vi "sub_ofdm_subcarrier_allocator.vi"(8 "fft size":i32=256, 9 "pilot symbol":cdb[](array[numeric]), 11 "message symbol":cdb[](array[numeric])) -> (3 "OFDM symbol":cdb[](array[numeric]))   [LabVIEW 2014]
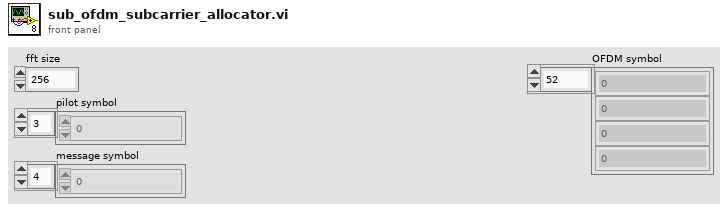
[diagram p1: front panel]
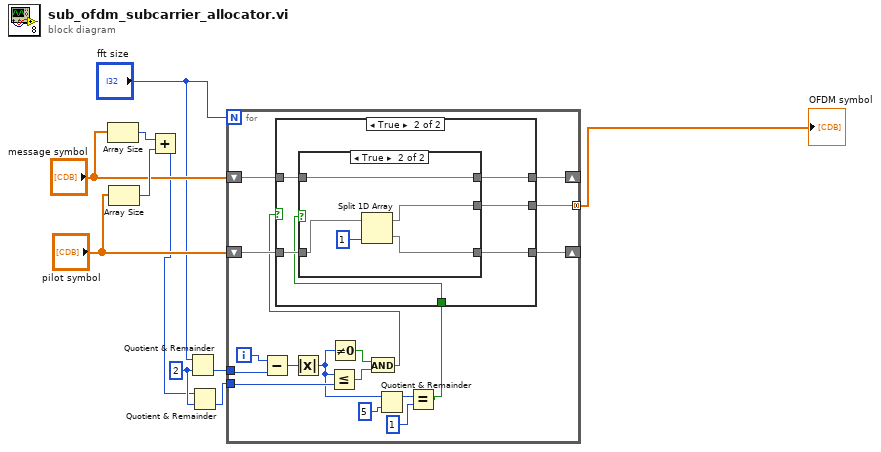
[diagram p0: block diagram]
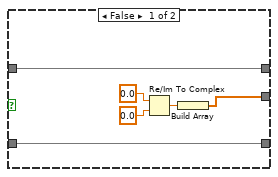
[diagram p2: hidden frame]
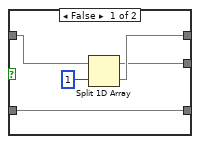
[diagram p3: hidden frame]
diagram:
  w3 = 2
  n1 = Array Size(array="message symbol") -> (size(s)=w10:i32)
  n2 = Array Size(array="pilot symbol") -> (size(s)=w9:i32)
  n3 = Add(x=w10, y=w9) -> (x+y=w2:i32)
  n4 = Quotient & Remainder(x="fft size", y=w3) -> (floor(x/y)=w5:i32)  [unwired: 1 out]
  n5 = Quotient & Remainder(x=w2, y=w3) -> (floor(x/y)=w1:i32)  [unwired: 1 out]
  n6 = for {
    N: "fft size" -> [_]
    shift-right: [w26] -> _
    shift-left: "pilot symbol" -> [w27]
    shift-right: [w20] -> _
    shift-left: "message symbol" -> [w25]
    tunnel: [w24] -> w4 mode=concatenating
    tunnel: w5 -> [w22]
    tunnel: w1 -> [w19]
    i -> [w23]
    n7 = Subtract(x=w23, y=w22) -> (x-y=w21:i32)
    n8 = Absolute Value(x=w21) -> (abs(x)=w15:i32)
    n9 = Less Or Equal?(x=w15, y=w19) -> (x <= y?=w17:bool)
    n10 = Not Equal To 0?(x=w15) -> (x != 0?=w18:bool)
    n11 = And(x=w18, y=w17) -> (x .and. y?=w16:bool)
    n12 = Quotient & Remainder(x=w15, y=5) -> (x-y*floor(x/y)=w13:i32)  [unwired: 1 out]
    n13 = Equal?(x=w13, y=1) -> (x = y?=w12:bool)
    n14 = case shown="True" w16 {
      tunnel: w27 -> [w32 w39]
      tunnel: [w32 w38] -> w26
      tunnel: w25 -> [w33 w37]
      tunnel: [w28 w36] -> w24
      tunnel: [w33 w35] -> w20
      tunnel: w12 -> [_ w34]
      frame False {
        n15 = Re/Im To Complex(1:0.0, 2:0.0) -> (0:w29:cdb)
        n16 = Build Array(w29) -> (w28:cdb[])
      }
      frame True {
        n17 = case shown="True" w34 {
          tunnel: w39 -> [w44 w49]
          tunnel: [w44 w47] -> w38
          tunnel: w37 -> [w43 w46]
          tunnel: [w42 w46] -> w35
          tunnel: [w40 w45] -> w36
          frame False {
            n18 = Split 1D Array(array=w43, index=1) -> (first subarray=w40:cdb[], second subarray=w42:cdb[])
          }
          frame True {
            n19 = Split 1D Array(array=w49, index=1) -> (first subarray=w45:cdb[], second subarray=w47:cdb[])
          }
        }
      }
    }
  }
  "OFDM symbol" <- w4
